vi "Convert to Excel.vi"(8 "error in (no error)":errorcluster, 10 "Path to TDMS/TDM File":path, 11 "Logging in":refnum<class "Logging.lvclass">) -> (0 "error out":errorcluster, 3 "Logging out":refnum<class "Logging.lvclass">)   [LabVIEW 2020, in "Logging.lvlib" / "Logging.lvclass"]
uses:
  Logging.lvclass
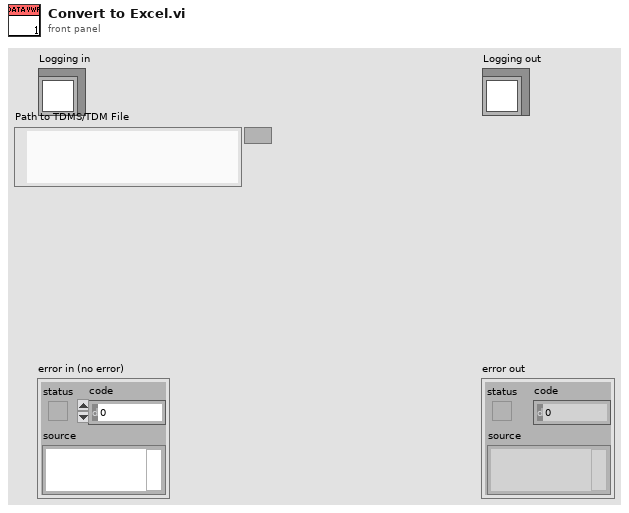
[diagram p1: front panel]
types:
  T1 = enum16{"open", "replace", "create", "open or create", "replace or create", "replace or create with confirmation"}
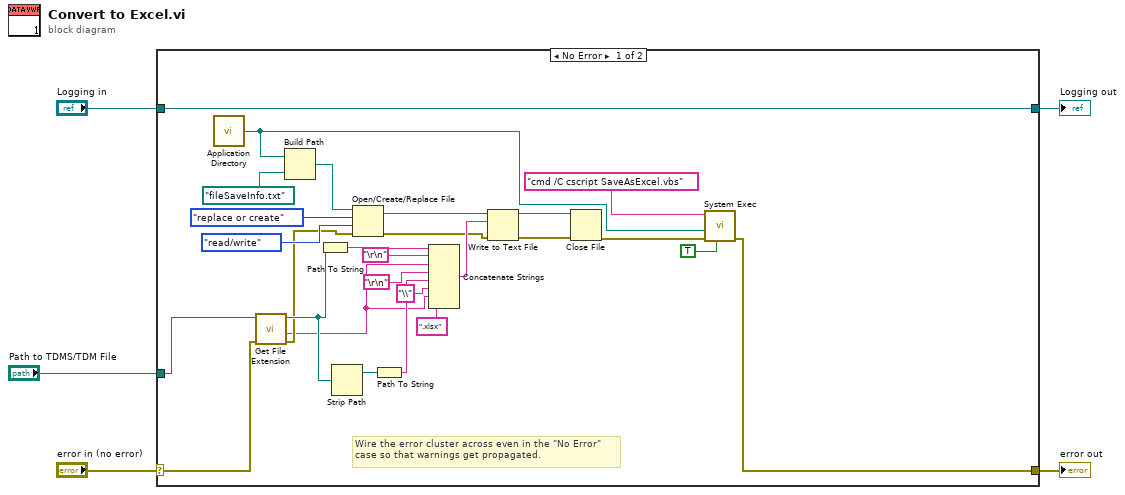
[diagram p0: block diagram]
diagram:
  n1 = case shown="No Error" "error in (no error)" {
    selector: "error in (no error)" -> [w12 w34]
    tunnel: [w11 w34] -> w4
    tunnel: [w32 w33] -> w2
    tunnel: "Logging in" -> [w32 w33]
    tunnel: "Path to TDMS/TDM File" -> [w26 _]
    frame No Error {
      # "Wire the error cluster across even in the \"No Error\"\ncase so that warnings get propagated."
      n2 = call <vilib>:"Application Directory.vi"() -> ("Application Directory"=w7:path)
      n3 = call <vilib>:"Get File Extension.vi"("error in (no error)"=w12, "file"=w26) -> ("error out"=w15:errorcluster, "filename without extension"=w10:string, "dup file"=w22:path)  [unwired: 5 in, 2 out]
      n4 = Build Path(base path=w7, name or relative path=path "fileSaveInfo.txt") -> (appended path=w30:path)
      n5 = Path To String(path=w22) -> (string=w25:string)
      n6 = Strip Path(path=w22) -> (stripped path=w21:path)  [unwired: 1 out]
      n7 = Open/Create/Replace File(file path (use dialog)=w30, error in=w15, operation (0:open)=T1."replace or create", access (0:read/write)=enum16{"read/write", "read-only", "write-only"}."read/write") -> (refnum out=w28:refnum<file>, error out=w16:errorcluster)  [unwired: 2 in, 1 out]
      n8 = Path To String(path=w21) -> (string=w20:string)
      n9 = Concatenate Strings(w25, "\r\n", w10, "\r\n", w20, "\\" ("string"), w10, ".xlsx" ("string")) -> (w19:string)
      n10 = Write to Text File(file (use dialog)=w28, text=w19, error in=w16) -> (refnum out=w18:refnum<file>, error out=w17:errorcluster)  [unwired: 1 in, 1 out]
      n11 = Close File(refnum=w18, error in=w17) -> (error out=w13:errorcluster)  [unwired: 1 out]
      n12 = call <vilib>:"System Exec.vi"("run minimized? (F)"=TRUE, "error in (no error)"=w13, "working directory"=w7, "command line"="cmd /C cscript SaveAsExcel.vbs") -> ("error out"=w11:errorcluster)  [unwired: 4 in, 3 out]
    }
    frame Error {
    }
  }
  "error out" <- w4
  "Logging out" <- w2
